vi "Siglent SDG X Series Arbitrary Waveform.vi"() -> ()   [LabVIEW 2022 SP3]
doc: "This example shows how to create then configure an arbitrary waveform."
uses:
  Siglent SDG X Series.lvlib
panel:
  in  "Disable Button":bool
  in  "Waveform Function (0: Sine)":u16(ring) items=["Sine", "Square", "Ramp", "DC", "Pulse", "Arb"]
  in  "Load Waveform Button":bool
  in  "VISA resource name":refnum<visa-resource-name>
  in  "DC Offset (0.00 V)":dbl
  in  "Frequency (1000 Hz)":dbl=1000.0 format="%#.6g"
  in  "Amplitude (1.0 Vpp)":dbl=1.0 format="%#.3f"
  in  "Channel (1:Channel 1)":i32(ring)=1 items=["Channel 1"=1, "Channel 2"=2]
  in  "Arbitrary Waveform Name":string="ARB1"
  # "(c) 2017 SIGLENT TECHNOLOGIES CO.,LTD. ALL RIGHTS RESERVED."
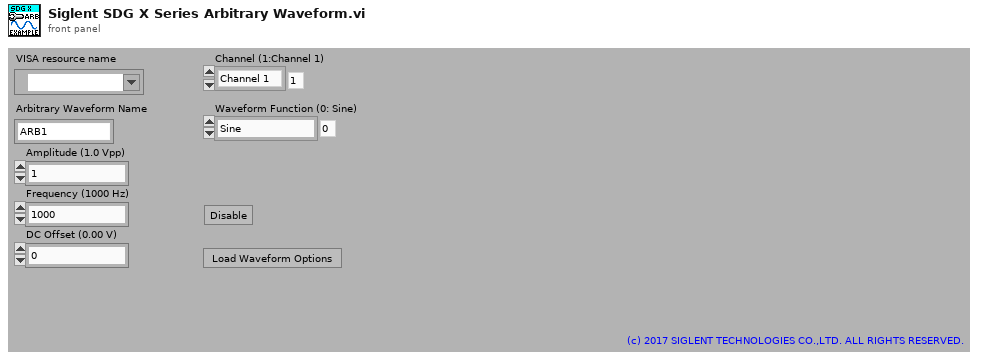
[diagram p1: front panel]
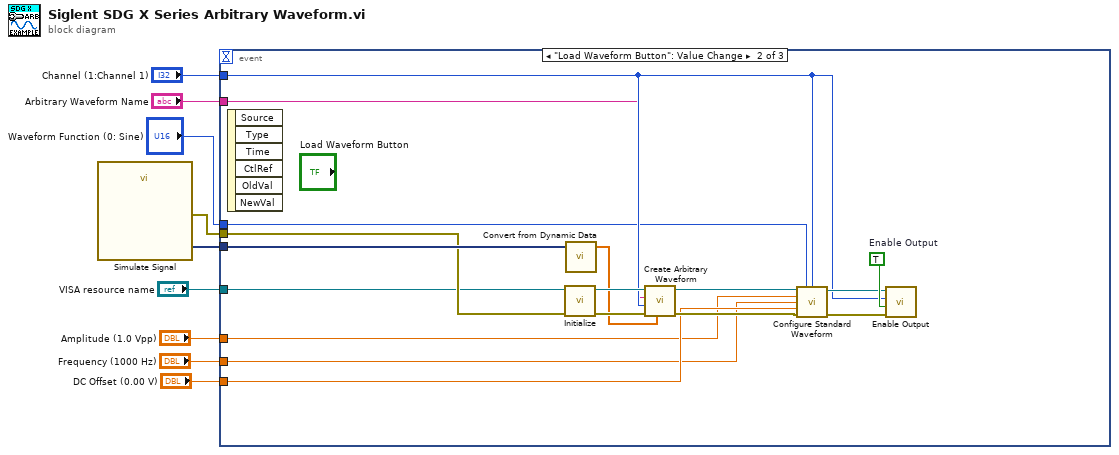
[diagram p0: block diagram]
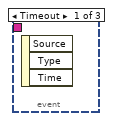
[diagram p2: hidden frame]
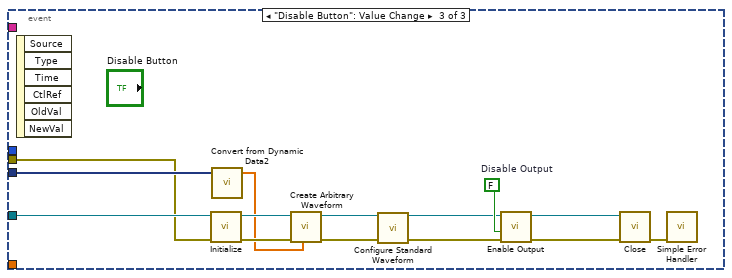
[diagram p3: hidden frame]
diagram:
  n1 = call "Simulate Signal"() -> ("正弦"=w7:dynamicdata, "error out"=w6:errorcluster)  [unwired: 14 in]
  n2 = event shown="[1] \"Load Waveform Button\": Value Change" {
    selector: _ -> [_ _ _]
    dyn-events: _ -> [_ _ _]
    timeout: _ -> [_ _ _]
    tunnel: "Channel (1:Channel 1)" -> [_ w18 _]
    tunnel: "Arbitrary Waveform Name" -> [_ w17 _]
    tunnel: w7 -> [_ w16 w29]
    tunnel: w6 -> [_ w15 w27]
    tunnel: "VISA resource name" -> [_ w14 w28]
    tunnel: "DC Offset (0.00 V)" -> [_ w13 _]
    tunnel: "Frequency (1000 Hz)" -> [_ w12 _]
    tunnel: "Amplitude (1.0 Vpp)" -> [_ w11 _]
    tunnel: "Waveform Function (0: Sine)" -> [_ w10 _]
    event Timeout {
      n3 = event-data() -> ()  [unwired: 1 in, 3 out]
    }
    event "Load Waveform Button": Value Change {
      w24 = TRUE  # Enable Output
      n4 = event-data() -> ()  [unwired: 1 in, 6 out]
      n5 = call "Initialize.vi"("error in (no error)"=w15, "VISA resource name"=w14) -> ("error out"=w26:errorcluster, "VISA resource name out"=w25:refnum<visa-resource-name>)  [unwired: 8 in]
      n6 = call "Convert from Dynamic Data"("Dynamic Data Type"=w16) -> ("Array"=w19:dbl[])  [unwired: 3 in]
      n7 = call "Create Arbitrary Waveform.vi"("Arbitrary Numeric Waveform Data"=w19, "error in (no error)"=w26, "Select Channel (1:Channel 1)"=w18, "Waveform Name (\"wave1\")"=w17, "VISA resource name"=w25) -> ("error out"=w21:errorcluster, "VISA resource name out"=w23:refnum<visa-resource-name>)  [unwired: 5 in]
      n8 = call "Configure Standard Waveform.vi"("VISA resource name"=w23, "Waveform Function (0: Sine)"=w10, "Channel (1:Channel 1)"=w18, "Amplitude (1.0 Vpp)"=w11, "Frequency (1000 Hz)"=w12, "DC Offset (0.00 V)"=w13, "error in (no error)"=w21) -> ("VISA resource name out"=w22:refnum<visa-resource-name>, "error out"=w20:errorcluster)  [unwired: 7 in]
      n9 = call "Enable Output.vi"("error in (no error)"=w20, "Enable Output (T: Enable)"=w24, "Channel (1:Channel 1)"=w18, "VISA resource name"=w22) -> ()  [unwired: 6 in, 2 out]
    }
    event "Disable Button": Value Change {
      w39 = FALSE  # Disable Output
      n10 = event-data() -> ()  [unwired: 1 in, 6 out]
      n11 = call "Initialize.vi"("error in (no error)"=w27, "VISA resource name"=w28) -> ("error out"=w34:errorcluster, "VISA resource name out"=w33:refnum<visa-resource-name>)  [unwired: 8 in]
      n12 = call "Convert from Dynamic Data2"("Dynamic Data Type"=w29) -> ("Array"=w32:dbl[])  [unwired: 3 in]
      n13 = call "Create Arbitrary Waveform.vi"("Arbitrary Numeric Waveform Data"=w32, "error in (no error)"=w34, "VISA resource name"=w33) -> ("error out"=w31:errorcluster, "VISA resource name out"=w30:refnum<visa-resource-name>)  [unwired: 7 in]
      n14 = call "Configure Standard Waveform.vi"("VISA resource name"=w30, "error in (no error)"=w31) -> ("VISA resource name out"=w36:refnum<visa-resource-name>, "error out"=w35:errorcluster)  [unwired: 12 in]
      n15 = call "Enable Output.vi"("error in (no error)"=w35, "Enable Output (T: Enable)"=w39, "VISA resource name"=w36) -> ("error out"=w37:errorcluster, "VISA resource name out"=w38:refnum<visa-resource-name>)  [unwired: 7 in]
      n16 = call "Close.vi"("error in (no error)"=w37, "VISA resource name"=w38) -> ("error out"=w40:errorcluster)  [unwired: 9 in]
      n17 = call <vilib>:"Simple Error Handler.vi"("error in (no error)"=w40) -> ()  [unwired: 4 in, 5 out]
    }
  }
